vi "example_get_device_polarity.vi"() -> ()   [LabVIEW 2012]
doc: "EXAMPLE: Get Device Polarity\n\nThis example VI retrieves the device's current polarity settings. \n\nProduced By:\n\nChristopher Lemieux\nKod Integrations, LLC\n4835 Marianne Drive\nMount Airy, MD 21771\nhttp://www.kodintegrations.com\nemail: clemieux@kodintegrations.com\nphone: (240) 687-1288"
uses:
  support/controls/polarity_item_group.ctl
  support/controls/polarity_items.ctl
panel:
  out "polarity_items":T1[](array[typedef])
  in  "device_index (def=0)":i32
  out "error out":errorcluster
  in  "error in (no error)":errorcluster
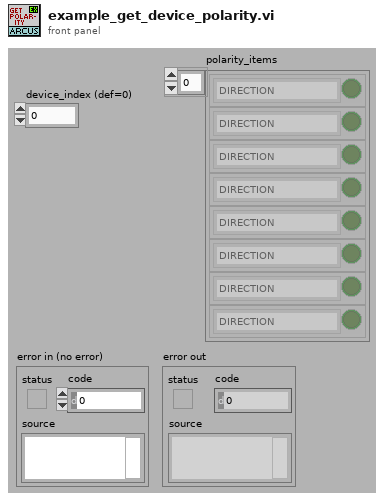
[diagram p1: front panel]
types:
  T1 = typedef "polarity_item_group.ctl" = cluster{"item":T2, "status":bool}
  T2 = typedef "polarity_items.ctl" = enum16{"DIRECTION", "LIMIT", "HOME", "DIG_OUT", "DIG_IN", "ENABLE_OUT", "JUMP_ERR"}
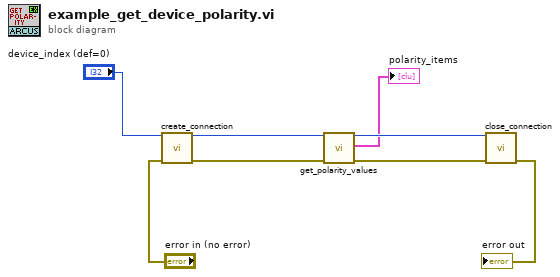
[diagram p0: block diagram]
diagram:
  n1 = call "create_connection.vi"("device_index (def=0)"="device_index (def=0)", "error in (no error)"="error in (no error)") -> ("reference"=w4:i32, "error out"=w5:errorcluster)  [unwired: 12 in]
  n2 = call "get_polarity_values.vi"("reference (in)"=w4, "error in (no error)"=w5) -> ("reference (dup)"=w3:i32, "polarity_items"=→"polarity_items":T1[], "error out"=w2:errorcluster)  [unwired: 14 in, 1 out]
  n3 = call "close_connection.vi"("reference"=w3, "error in (no error)"=w2) -> ("error out"=→"error out":errorcluster)  [unwired: 13 in]
